vi "Event Handle Loop_Draw_Direction Button.vi"(8 "error in (no error)":errorcluster, 10 "Picture In":picture, 11 "QMenu Class in":refnum<class "QMenu Class.lvclass">) -> (0 "error out":errorcluster, 2 "Picture Out":picture, 3 "QMenu Class out":refnum<class "QMenu Class.lvclass">)   [LabVIEW 2020, in "QTab.lvlib" / "QMenu Class.lvclass"]
uses:
  QMenu Class.lvclass
  QMenu Class.lvclass/QMenu Class.ctl
  Read Left Button Image.vi
  Read Right Button Image.vi
  Read Total Button Count.vi
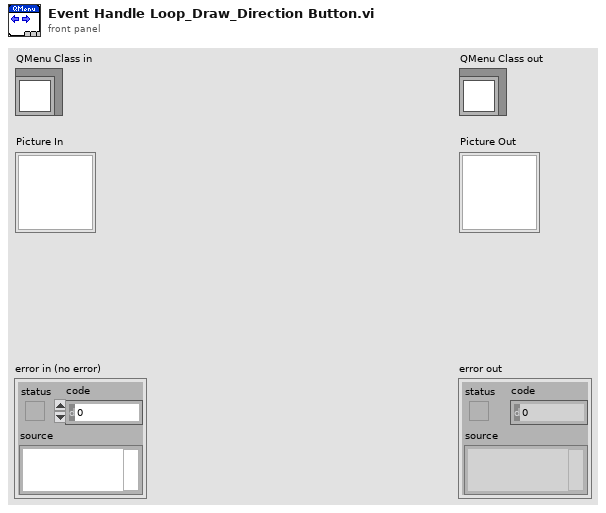
[diagram p1: front panel]
types:
  T1 = typedef "imagedata.ctl" = cluster{"image type":i32, "image depth":i32, "image":u8[], "mask":u8[], "colors":u32[], "Rectangle":cluster{"left":i16, "top":i16, "right":i16, "bottom":i16}}
  T2 = cluster{"left":i16, "top":i16, "right":i16, "bottom":i16}
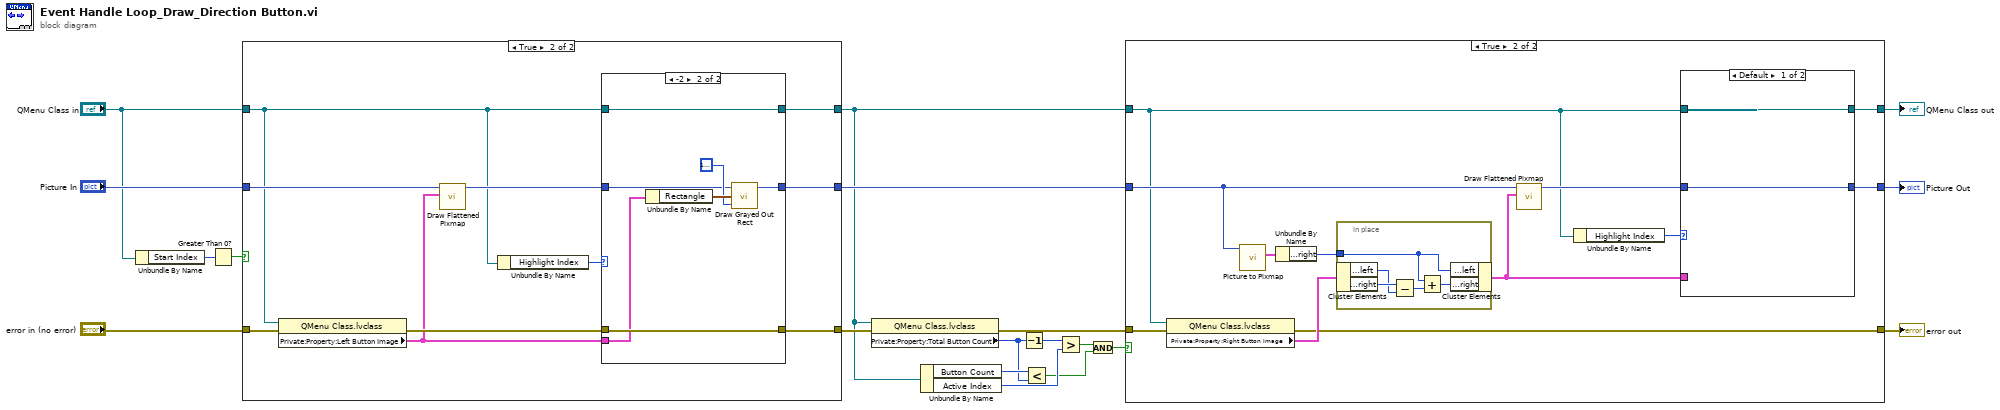
[diagram p0: block diagram]
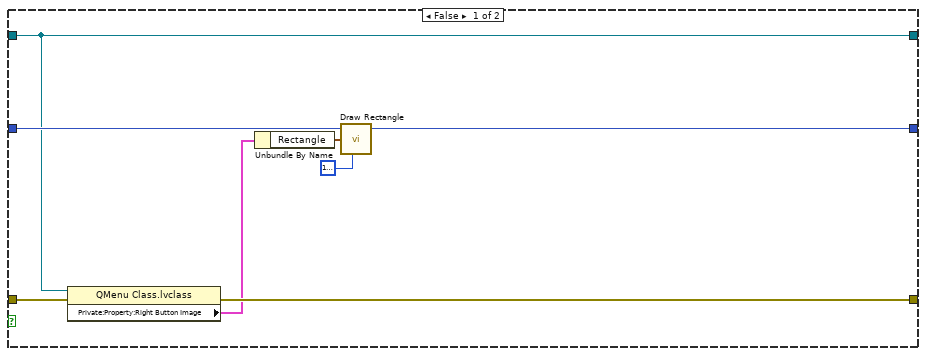
[diagram p2: hidden frame]
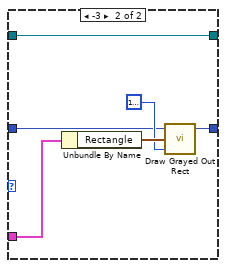
[diagram p3: hidden frame]
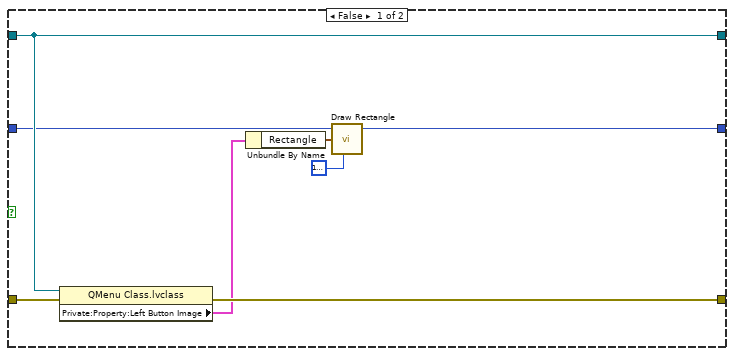
[diagram p4: hidden frame]
diagram:
  n1 = Unbundle By Name("QMenu Class in") -> ("Start Index"=w12:i32)
  n2 = Greater Than 0?(x=w12) -> (x > 0?=w7:bool)
  n3 = case shown="True" w7 {
    tunnel: "error in (no error)" -> [w27 w37]
    tunnel: [w23 w35] -> w11
    tunnel: "Picture In" -> [w25 w34]
    tunnel: [w24 w31] -> w17
    tunnel: [w26 w29] -> w9
    tunnel: "QMenu Class in" -> [w26 w28]
    frame False {
      n4 = property class="QMenu Class.lvclass"(reference=w26, error in=w27) -> (error out=w23:errorcluster, "Private:Property:Left Button Image"=w22:T1)  [unwired: 1 out]
      n5 = Unbundle By Name(w22) -> ("Rectangle"=w21:T2)
      n6 = call <vilib>:"Draw Rectangle.vi"("picture"=w25, "rect"=w21, "color(black)"=u32 16777216) -> ("new picture"=w24:picture)  [unwired: 6 in]
    }
    frame True {
      n7 = property class="QMenu Class.lvclass"(reference=w28, error in=w37) -> (error out=w33:errorcluster, "Private:Property:Left Button Image"=w32:T1)  [unwired: 1 out]
      n8 = call <vilib>:"Draw Flattened Pixmap.vi"("image data"=w32, "picture"=w34) -> ("new picture"=w36:picture)  [unwired: 7 in]
      n9 = Unbundle By Name(w28) -> ("Highlight Index"=w30:i32)
      n10 = case shown="-2" w30 {
        tunnel: w32 -> [_ w42]
        tunnel: w33 -> [w38 w46]
        tunnel: w36 -> [w39 w43]
        tunnel: w28 -> [w40 w47]
        tunnel: [w40 w47] -> w29
        tunnel: [w38 w46] -> w35
        tunnel: [w39 w41] -> w31
        frame Default {
        }
        frame -2 {
          n11 = Unbundle By Name(w42) -> ("Rectangle"=w45:T2)
          n12 = call <vilib>:"Draw Grayed Out Rect.vi"("color(black)"=u32 16777225, "rect"=w45, "picture"=w43) -> ("new picture"=w41:picture)  [unwired: 2 in]
        }
      }
    }
  }
  n13 = property class="QMenu Class.lvclass"(reference=w9, error in=w11) -> (error out=w10:errorcluster, "Private:Property:Total Button Count"=w4:i32)  [unwired: 1 out]
  n14 = Unbundle By Name(w9) -> ("Button Count"=w5:i32, "Active Index"=w8:i32)
  n15 = Decrement(x=w4) -> (x-1=w6:i32)
  n16 = Less?(x=w5, y=w4) -> (x < y?=w2:bool)
  n17 = Greater?(x=w6, y=w8) -> (0:w3:bool)
  n18 = And(x=w3, y=w2) -> (x .and. y?=w1:bool)
  n19 = case shown="True" w1 {
    tunnel: w17 -> [w53 w65]
    tunnel: [w51 w61] -> w16
    tunnel: [w48 w60] -> w15
    tunnel: [w50 w56] -> w14
    tunnel: w10 -> [w52 w58]
    tunnel: w9 -> [w51 w57]
    frame False {
      n20 = property class="QMenu Class.lvclass"(reference=w51, error in=w52) -> (error out=w50:errorcluster, "Private:Property:Right Button Image"=w49:T1)  [unwired: 1 out]
      n21 = Unbundle By Name(w49) -> ("Rectangle"=w55:T2)
      n22 = call <vilib>:"Draw Rectangle.vi"("picture"=w53, "rect"=w55, "color(black)"=u32 16777216) -> ("new picture"=w48:picture)  [unwired: 6 in]
    }
    frame True {
      n23 = property class="QMenu Class.lvclass"(reference=w57, error in=w58) -> (error out=w56:errorcluster, "Private:Property:Right Button Image"=w67:T1)  [unwired: 1 out]
      n24 = call <vilib>:"Picture to Pixmap.vi"("picture"=w65) -> ("image data"=w64:T1)  [unwired: 9 in, 1 out]
      n25 = Unbundle By Name(w64) -> ("Rectangle.right"=w66:i16)
      n26 = in-place {
        in-place-border: w66 -> [w76]
        n27 = in-place-cluster #1(w67) -> ("Rectangle.left"=w79:i16, "Rectangle.right"=w80:i16)
        n28 = Subtract(x=w80, y=w79) -> (x-y=w78:i16)
        n29 = Add(x=w76, y=w78) -> (x+y=w77:i16)
        n30 = in-place-cluster #1("Rectangle.left"=w76, "Rectangle.right"=w77) -> (w59:T1)
      }
      n31 = call <vilib>:"Draw Flattened Pixmap.vi"("image data"=w59, "picture"=w65) -> ("new picture"=w62:picture)  [unwired: 7 in]
      n32 = Unbundle By Name(w57) -> ("Highlight Index"=w63:i32)
      n33 = case shown="Default" w63 {
        tunnel: w59 -> [_ w71]
        tunnel: w62 -> [w68 w72]
        tunnel: w57 -> [w69 w75]
        tunnel: [w69 w75] -> w61
        tunnel: [w68 w70] -> w60
        frame Default {
        }
        frame -3 {
          n34 = Unbundle By Name(w71) -> ("Rectangle"=w74:T2)
          n35 = call <vilib>:"Draw Grayed Out Rect.vi"("color(black)"=u32 16777225, "rect"=w74, "picture"=w72) -> ("new picture"=w70:picture)  [unwired: 2 in]
        }
      }
    }
  }
  "error out" <- w14
  "QMenu Class out" <- w16
  "Picture Out" <- w15
